vi "VISubPanelRemove.vi"(4 "'Stop' Value":variant, 5 "Remove? [T]":bool=TRUE, 6 "'Stop' Label":string="Stop", 7 "SubPanel in":refnum<vi>, 8 "error in (no error)":errorcluster, 9 "TimeOut (ms) [-1]":i32=-1) -> (0 "error out":errorcluster, 1 "Timed Out?":bool)   [LabVIEW 2020]
doc: "This VI will remove the loaded _Cluster.vi from the subpanel"
uses:
  CtlReferences.lvclass/CtlReferences.ctl
  CtlReferences.lvclass
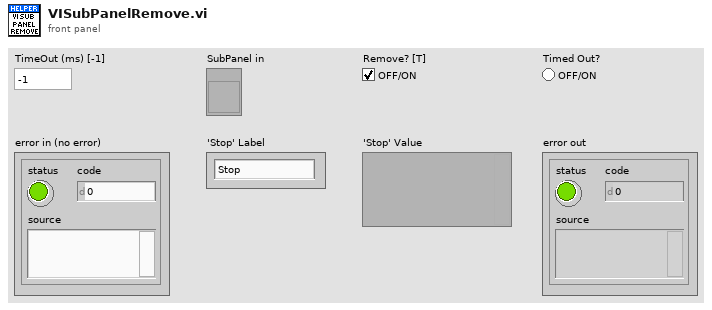
[diagram p1: front panel]
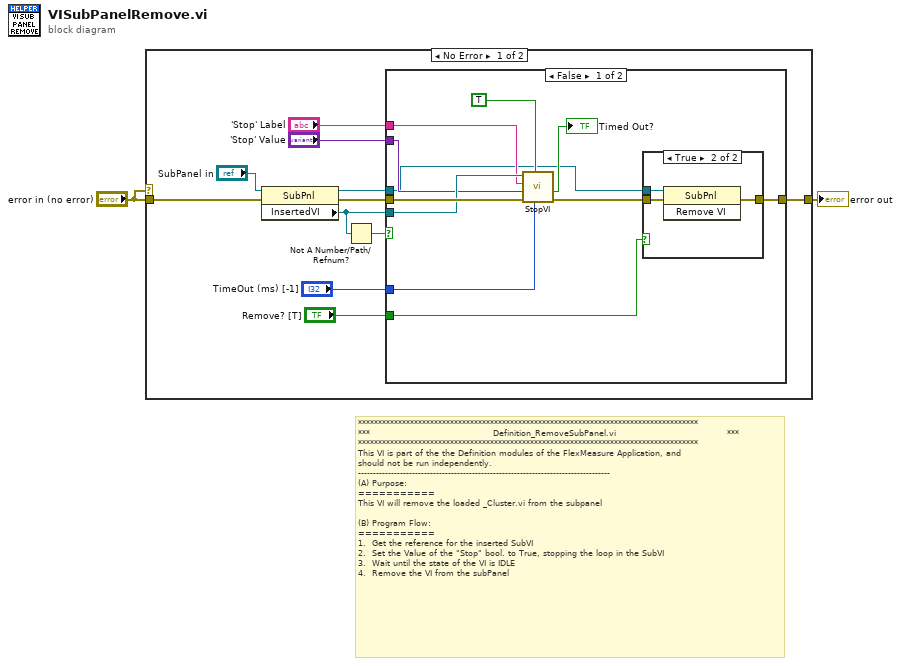
[diagram p0: block diagram]
diagram:
  # "*************************************************************************************\n***                                         Definition_RemoveSubPanel.vi                                     ***\n*************************************************************************************\nThis VI is part of the the Definition modules of the FlexMeasure Application, and \nshould not be run independently.\n------------------------------------------------------------------------------------\n(A) Purpose:\n===========\nThis VI will remove the loaded _Cluster.vi from the subpanel\n\n(B) Program Flow:\n===========\n1.  Get the reference for the inserted SubVI\n2.  Set the Value of the \"Stop\" bool. to True, stopping the loop in the SubVI\n3.  Wait until the state of the VI is IDLE\n4.  Remove the VI from the subPanel"
  n1 = case shown="No Error" "error in (no error)" {
    tunnel: "error in (no error)" -> [w10 w30]
    tunnel: [w11 w30] -> w2
    frame No Error {
      n2 = property class="SubPnl"(reference="SubPanel in", error in=w10) -> (reference out=w13:refnum<vi>, error out=w9:errorcluster, "InsertedVI"=w8:refnum<vi>)
      n3 = Not A Number/Path/Refnum?(number/path/refnum=w8) -> (NaN/Path/Refnum?=w7:bool)
      n4 = case shown="False" w7 {
        tunnel: w13 -> [w15 _]
        tunnel: [w24 w29] -> w11
        tunnel: w9 -> [w23 w29]
        tunnel: w8 -> [w22 _]
        tunnel: "TimeOut (ms) [-1]" -> [w18 _]
        tunnel: "'Stop' Label" -> [w17 _]
        tunnel: "'Stop' Value" -> [w16 _]
        tunnel: "Remove? [T]" -> [w14 _]
        frame False {
          n5 = call "StopVI.vi"("TimeOut (ms) [-1]"=w18, "ForceClose"=TRUE, "error in (no error)"=w23, "'Stop' Value"=w16, "'Stop' Label"=w17, "VI Reference"=w22) -> ("error out"=w19:errorcluster, "Timed Out?"=→"Timed Out?":bool)  [unwired: 3 in, 1 out]
          n6 = case shown="True" w14 {
            tunnel: w15 -> [_ w28]
            tunnel: w19 -> [w25 w27]
            tunnel: [w25 w26] -> w24
            frame False {
            }
            frame True {
              n7 = invoke class="SubPnl" method="Remove VI"(reference=w28, error in=w27) -> (error out=w26:errorcluster)  [unwired: 1 in, 2 out]
            }
          }
        }
        frame True {
        }
      }
    }
    frame Error {
    }
  }
  "error out" <- w2
